vi "CRYASIOExit.vi"(11 "error in (no error)":errorcluster) -> (0 "bResult":bool, 3 "error out":errorcluster)   [LabVIEW 2013]
uses:
  CRYASIO Global.vi
  CRY_ASIO.dll
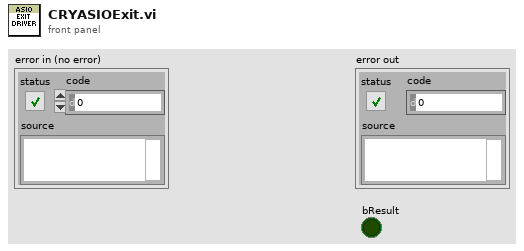
[diagram p1: front panel]
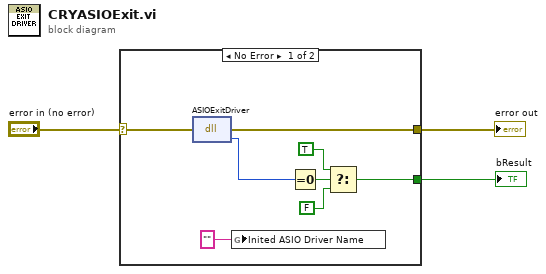
[diagram p0: block diagram]
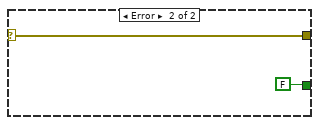
[diagram p2: hidden frame]
diagram:
  n1 = case shown="No Error" "error in (no error)" {
    selector: "error in (no error)" -> [w7 w13]
    tunnel: [w6 w13] -> w2
    tunnel: [w8 FALSE] -> w1
    frame No Error {
      n2 = dll-call lib="D:/LabView_Project/CRY6181/CRY_ASIO.dll" fn="ASIOExitDriver"(error in=w7) -> (error out=w6:errorcluster, "return type"=w5:i32)  [unwired: 2 in, 1 out]
      n3 = global write "CRYASIO Global.vi" "Inited ASIO Driver Name"("" ("Inited ASIO Driver Name")) -> ()
      n4 = Equal To 0?(x=w5) -> (x = 0?=w11:bool)
      n5 = Select(t=TRUE, s=w11, f=FALSE) -> (s? t:f=w8:bool)
    }
    frame Error {
    }
  }
  "error out" <- w2
  "bResult" <- w1
